vi "Day3-1.vi"() -> ()   [LabVIEW 2021]
panel:
  out "sum":i32
  out "Array 2":i32[](array[numeric])
  out "Array":string[](array[string])
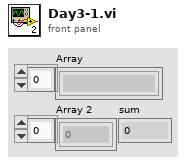
[diagram p1: front panel]
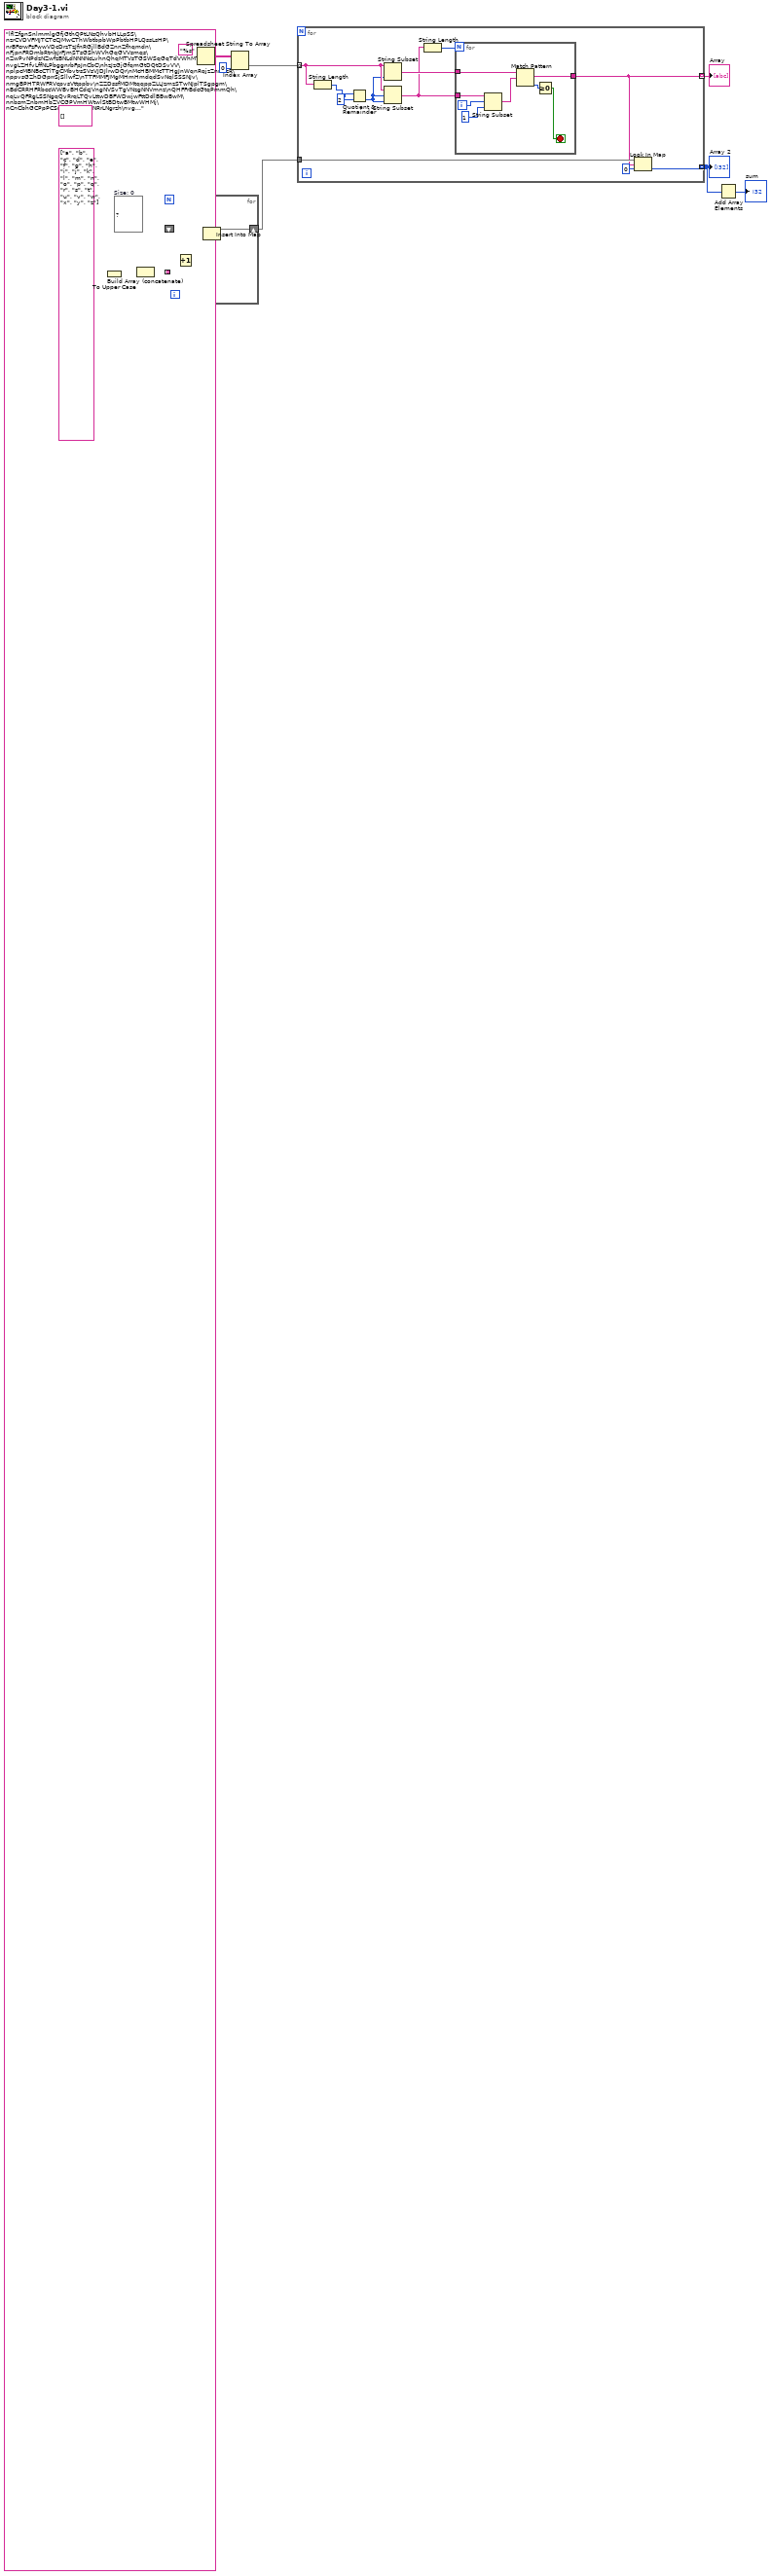
[diagram p0: block diagram]
diagram:
  w6 = map{string, i32} {}  # Size: 0
  w8 = string[] ["a", "b", "c", "d", "e", "f", "g", "h", "i", "j", "k", "l", "m", "n", "o", "p", "q", "r", "s", "t", "u", "v", "w", "x", "y", "z"]
  n1 = To Upper Case(1:w8) -> (0:w9:string[])
  n2 = Build Array (concatenate)(w8, w9) -> (w7:string[])
  n3 = for {
    tunnel: w7 -> [w18] mode=indexing
    shift-right: [w15] -> w4
    shift-left: w6 -> [w19]
    i -> [w17]
    n4 = Increment(x=w17) -> (x+1=w16:i32)
    n5 = Insert Into Map(map in=w19, key=w18, value=w16) -> (map out=w15:map{string, i32})  [unwired: 2 out]
  }
  n6 = Spreadsheet String To Array(format string="%s", spreadsheet string="lflZfgnSnlmmlgGfjGthQPtLNsQhvbHLLpSS\nzrCVDVFMJTCTcCJMwCThWbtbpbWpPbtbHPLQssLsHP\nrBFcrwFzFwwVDcDrzTzJfnRGjllBdGZnnZfhqmdn\nFjpnFRDmbRtnbJrFJmSTsGShWVhGqGVVsmqs\nZwPvNPdzNZwfzBNLdNNNNcLvhnQhqMTVsTGSWSqGqTdVWhMT\nvgLZHfvLffNLPbggnrbFpJnCbC\nhzJzGjGfqmGtDQtDSvVV\nplpcMBNBcCTlTgCMbvtrsSVsVJDJlrwDQr\nMcHBMMcTTHgJnWqnRqjzZnnRzR\nppvsGZhDGprrSjSllwfZ\nTTFMMFJMgMHmHmdqdSvNqlSSSNJv\nmgBPHTRWFRVcpvsVttppbv\nZZDssfMDMtqqppZLLJzmzSTwNJplTSgpgm\nBdCRRHFRbccWWBvBHCdcJVngNVSvTgVNzgNNVmnz\nQHFFrBdcGtqPmmQh\nqLvQFRgLSSNgqQvRrqLTQvLttwDBFWDwjwFttDdlBBwBwM\nnbsmZnbmHbZVCGPVmHWtwlStBDtwBMtwWHMj\nCnCbhGCPpPCSnZmrgRNRqNRrLNgrzh\nvg...", array type (2D Dbl)=string[][] []) -> (array=w11:string[][])  [unwired: 1 in]
  n7 = Index Array(array=w11, index (col)=0 ("disabled index (col)")) -> (element=w5:string[])  [unwired: 1 in]
  n8 = for {
    tunnel: w5 -> [w28] mode=indexing
    tunnel: w4 -> [w23]
    tunnel: [w21] -> w2 mode=indexing
    tunnel: [w20] -> w3 mode=indexing
    n9 = String Length(string=w28) -> (length=w30:i32)
    n10 = Quotient & Remainder(x=w30, y=2) -> (floor(x/y)=w27:i32)  [unwired: 1 out]
    n11 = String Subset(string=w28, length (rest)=w27) -> (substring=w26:string)  [unwired: 1 in]
    n12 = String Subset(string=w28, offset (0)=w27, length (rest)=w27) -> (substring=w24:string)
    n13 = String Length(string=w24) -> (length=w25:i32)
    n14 = for {
      N: w25 -> [_]
      tunnel: w26 -> [w38]
      tunnel: w24 -> [w36]
      tunnel: [w31] -> w20
      i -> [w35]
      stop <- w32 stop-if-true
      n15 = String Subset(string=w36, offset (0)=w35, length (rest)=1 ("length (rest)")) -> (substring=w34:string)
      n16 = Match Pattern(string=w38, regular expression=w34) -> (match substring=w31:string, offset past match=w33:i32)  [unwired: 1 in, 2 out]
      n17 = Greater Or Equal To 0?(x=w33) -> (x >= 0?=w32:bool)
    }
    n18 = Look In Map(map=w23, key=w20, default value=0) -> (value=w21:i32)  [unwired: 1 out]
  }
  "Array" <- w3
  "Array 2" <- w2
  n19 = Add Array Elements(numeric array=w2) -> (sum=→"sum":i32)
